vi "TestBsp.vi"() -> ()   [LabVIEW 2024]
uses:
  Downloads/Treiber/Treiber/Treiber Heizung/Thermostat Treiber.lvlib
panel:
  in  "stop":bool
  out "error out":errorcluster
  in  "error in (no error)":errorcluster
  in  "Ventilregler":dbl
  out "Temp":dbl
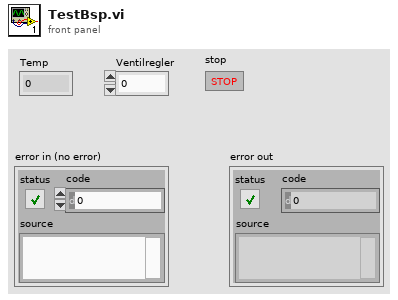
[diagram p1: front panel]
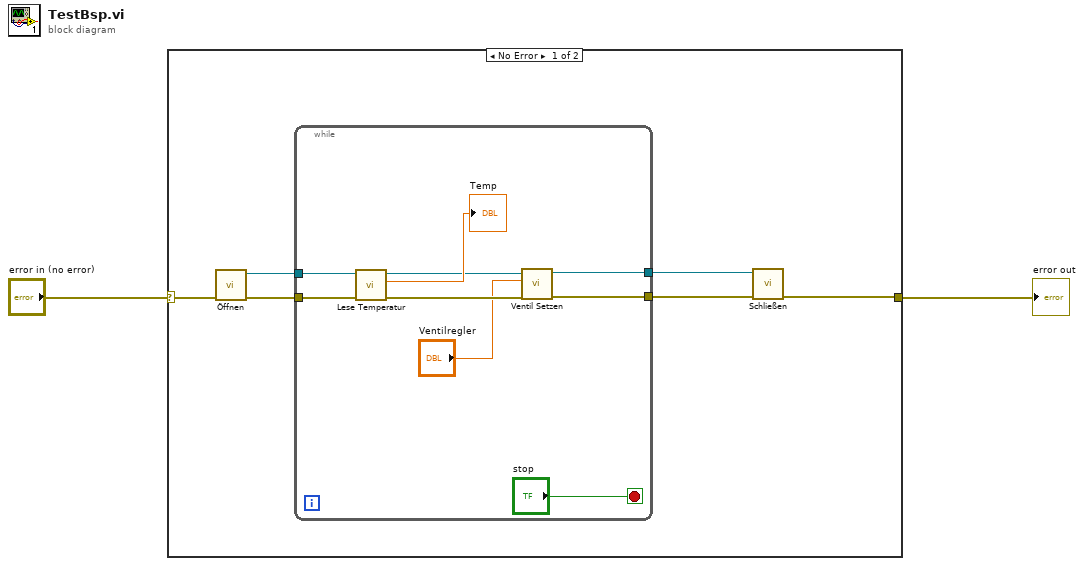
[diagram p0: block diagram]
diagram:
  n1 = case shown="No Error" "error in (no error)" {
    selector: "error in (no error)" -> [w8 w18]
    tunnel: [w3 w18] -> w1
    frame No Error {
      n2 = call "Öffnen.vi"("Error In"=w8) -> ("Error Out"=w7:errorcluster, "Verbindungs-ID"=w6:refnum<k16>)  [unwired: 9 in]
      n3 = while {
        tunnel: w7 -> [w16]
        tunnel: w6 -> [w17]
        tunnel: [w11] -> w5
        tunnel: [w10] -> w4
        stop <- "stop" stop-if-true
        n4 = call "Lese Temperatur.vi"("Error In"=w16, "Verbindungs-ID in"=w17) -> ("Error Out"=w13:errorcluster, "Temperatur"=→"Temp":dbl, "Verbindungs-ID out"=w14:refnum<k16>)  [unwired: 5 in, 2 out]
        n5 = call "Ventil Setzen.vi"("Error In"=w13, "Thermostat in %"="Ventilregler", "Verbindungs-ID in"=w14) -> ("Error Out"=w10:errorcluster, "Verbindungs-ID out"=w11:refnum<k16>)  [unwired: 7 in]
      }
      n6 = call "Schließen.vi"("Error In"=w4, "Verbindungs-ID"=w5) -> ("Error Out"=w3:errorcluster)  [unwired: 9 in]
    }
    frame Error {
    }
  }
  "error out" <- w1
